vi "StartAOVoltage_Audio.vi"(0 "Physical Channel(s)":tag="DAQ/ao0", 5 "Max Voltage":dbl=10.0, 7 "Min Voltage":dbl=-10.0, 9 "Parameters":T1={"Waveform Type"=0, "Desired Frequency"=1000.0, "Amplitude"=1.0, "Offset"=0.0} {"Waveform Type" items=[" Sine Wave", " Triangle Wave", " Square Wave", " Sawtooth Wave"]}) -> (15 "error out":errorcluster)   [LabVIEW 2012]
doc: "I. Description:\nThis example demonstrates how to continuously output a waveform using an internal sample clock. The output waveform will be stored on the on-board memory of the device and then generated continuously from there.\n\nII. Instructions for Running:\n1. Select the Physical Channel to correspond to where your signal is output on the DAQ device.\n2. Enter the Minimum and Maximum Voltage Ranges.\n3. Specify the Desired Frequency of the output Waveform\n4. Enter the Waveform Information. See the documentation of the Waveform Buffer Generation SubVI for information on each parameter.\nNOTE: Make sure the total number of samples contained in the Analog Output Waveform does not exceed the size of the on-board memory of the device.\n\n\nIII. Block Diagram Steps:\n1. Create an Analog Output Voltage Task\n2. Call the DAQmx Timing (Use Waveform) VI which sets the sample clock rate based on the input waveform parameters, and set the sample mode to Continuous.\n3. Configure the analog output operation to store the waveform on the on-board memory of the device.\n4. Write the waveform to the output buffer.\n5. Call the Start VI.\n6. Loop continuously until the user presses the Stop button. Check for errors every 100 ms using the Is Task Done? VI\n7. Call the Clear Task VI to clear the Task.\n8. Use the popup dialog box to display an error or warning if any.\n\nIV. I/O Connections Overview:\nMake sure your signal output terminal matches the Physical Channel I/O Control. For further connection information, refer to your hardware reference manual."
uses:
  <vilib>/DAQmx/write.llb/DAQmx Write (Analog 1D Wfm NChan NSamp).vi
  <vilib>/DAQmx/create/channels.llb/DAQmx Create Channel (AO-Voltage-Basic).vi
  <vilib>/DAQmx/configure/timing.llb/DAQmx Timing (Use Waveform).vi
  <vilib>/DAQmx/miscellaneous.llb/DAQmx Fill In Error Info.vi
  <resource>/objmgr/daqmx.rc
panel:
  in  "Sample Rate":dbl=96000.0
  out "Sample Rate":dbl
  out "dt":dbl
  out "Output Waveforms":waveform(dbl)[](graph) caption="Output Waveform"
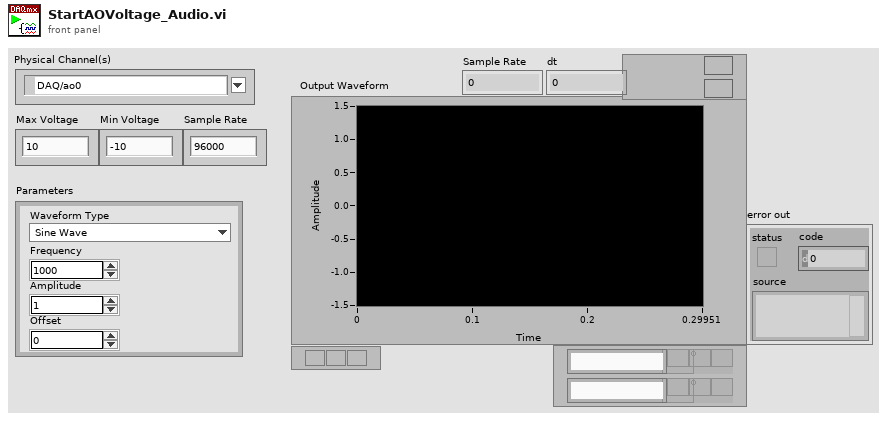
[diagram p1: front panel]
types:
  T1 = cluster{"Waveform Type":u16, "Desired Frequency":dbl, "Amplitude":dbl, "Offset":dbl}
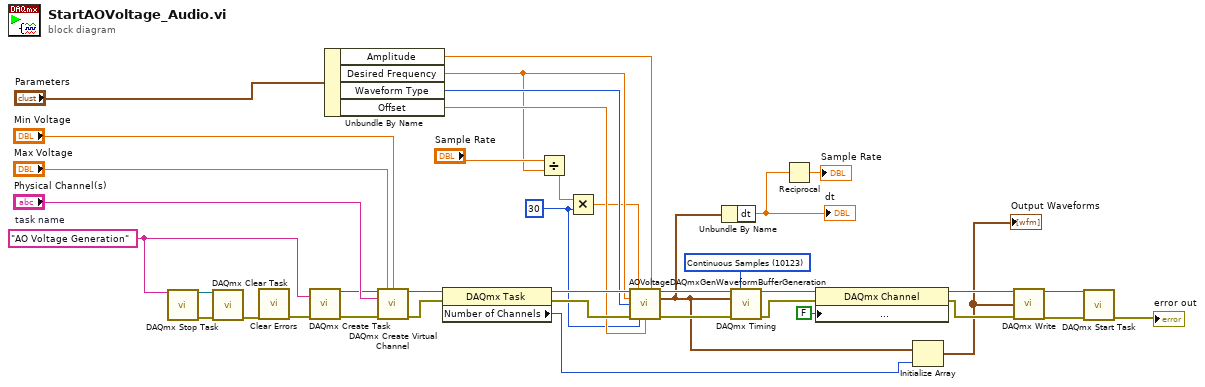
[diagram p0: block diagram]
diagram:
  w2 = 30
  w11 = "AO Voltage Generation"  # task name
  w23 = 10123 items=["Finite Samples"=10178, "Continuous Samples"=10123] ("sample mode")
  n1 = call <vilib>:"DAQmx Stop Task.vi"("task/channels in"=w11) -> ("task out"=w13:refnum<k21>, "error out"=w12:errorcluster)  [unwired: 13 in]
  n2 = call <vilib>:"DAQmx Clear Task.vi"("task in"=w13, "error in"=w12) -> ("error out"=w10:errorcluster)  [unwired: 13 in]
  n3 = call <vilib>:"Clear Errors.vi"("error in (no error)"=w10) -> ("error out"=w9:errorcluster)  [unwired: 6 in]
  n4 = call <vilib>:"DAQmx Create Task.vi"("new task name"=w11, "error in"=w9) -> ("task out"=w14:refnum<k21>, "error out"=w15:errorcluster)  [unwired: 12 in]
  n5 = Unbundle By Name("Parameters") -> ("Amplitude"=w33:dbl, "Desired Frequency"=w4:dbl, "Waveform Type"=w32:u16, "Offset"=w31:dbl)
  n6 = call-poly <vilib>:"DAQmx Create Virtual Channel.vi"("task in"=w14, "maximum value"="Max Voltage", "minimum value"="Min Voltage", "physical channels"="Physical Channel(s)", "error in"=w15) -> ("task out"=w16:refnum<k21>, "error out"=w27:errorcluster)  [unwired: 9 in]
  n7 = property class="DAQmx Task"(reference=w16, error in=w27) -> (reference out=w36:refnum<k21>, error out=w35:errorcluster, "Number of Channels"=w20:u32)
  n8 = Divide(x="Sample Rate", y=w4) -> (x/y=w3:dbl)
  n9 = Multiply(x=w3, y=w2) -> (x*y=w1:dbl)
  n10 = call "AOVoltageDAQmxGenWaveformBufferGeneration.vi"("task/channels in"=w36, "Samples per Buffer"=w1, "Amplitude"=w33, "Desired Frequency"=w4, "Waveform Type"=w32, "error in (no error)"=w35, "Cycles per Buffer"=w2, "Offset"=w31) -> ("task out"=w21:refnum<k21>, "Waveform"=w8:waveform(dbl), "error out"=w22:errorcluster)  [unwired: 3 in, 2 out]
  n11 = Unbundle By Name(w8) -> ("dt"=w7:dbl)
  "dt" <- w7
  n12 = call-poly <vilib>:"DAQmx Timing.vi"("task/channels in"=w21, "sample mode"=w23, "waveform"=w8, "error in"=w22) -> ("task out"=w25:refnum<k21>, "error out"=w26:errorcluster)  [unwired: 10 in]
  n13 = Reciprocal(x=w7) -> (1/x=→"Sample Rate":dbl)
  n14 = property class="DAQmx Channel"(reference=w25, error in=w26, "Analog Output:General Properties:Advanced:Data Transfer and Memory:Use Only Onboard Memory"=FALSE ("AO.UseOnlyOnBrdMem")) -> (reference out=w19:refnum<k21>, error out=w37:errorcluster)
  n15 = Initialize Array(w8, w20) -> (w18:waveform(dbl)[])
  "Output Waveforms" <- w18
  n16 = call-poly <vilib>:"DAQmx Write.vi"("task/channels in"=w19, "data"=w18, "error in"=w37) -> ("task out"=w39:refnum<k21>, "error out"=w38:errorcluster)  [unwired: 10 in, 1 out]
  n17 = call <vilib>:"DAQmx Start Task.vi"("task/channels in"=w39, "error in"=w38) -> ("error out"=→"error out":errorcluster)  [unwired: 12 in, 1 out]
